vi "Demo RGB LED - Chaser With R G B Alternate onboard LED.vi"   [LabVIEW 2015]
doc: "This example demonstrates a theater light chaser on a 1-wire RGB LED strip using a WS2811 or WS2812 controller. The color of all LEDs can be preset on the front panel as well as the number of lights to cycle in the light chase. The time delay can also be adjusted to change the dramatic effect."
uses:
  <vilib>/Aledyne-TSXperts/Arduino Compatible Compiler for LabVIEW/Code Generator/Arduino APIs/Digital/PinDirection.ctl
  <vilib>/Aledyne-TSXperts/Arduino Compatible Compiler for LabVIEW/Code Generator/Arduino APIs/RGB LED Strip/RGB Strip Mode.ctl
  LED State.vi
  <vilib>/Aledyne-TSXperts/Arduino Compatible Compiler for LabVIEW/Arduino Compatible Compiler for LabVIEW.lvlib
panel:
  # "Overview: Demonstrates a theater light chaser on a 1-wire RGB LED strip using a WS2811 or WS2812 controller.  The color of all LEDs can be preset as well as the number of lights to cycle in the light chase.  The time delay can also be adjusted to change the dramatic effect.\n\nInstructions:\n1. Wire a 1-wire LED strip to a digital pin on the Arduino board.  Follow wiring instructions from the manufacturer.  A 100-500 ohm resistor is usually recommended between the Arduino digital output and the LED strip's data in pin.  Also, a 100 uF capacitor between the ground and power input may reduce noise on from the power supply.  It is also recommended to power the LED strip from a separate power input if available on the strip.  When daisy chaining LED strips, it is recommended to only daisy chain the Data line and to power each strip from a separate power input.\n2. Set the Digital Pin wired below.\n3. Set the Mode to the correct setting for your LED strip (the WS2812 uses 800kHz GRB).\n4. Set the Number of LEDs on your strip.  This can be set to any number equal to or smaller than the number of physical LEDs on the strip of you do not wish to power up all of them.\n5. Set Chase Every N Pixel to adjust how many pixels are moved on every cycle.\n6. Set the delay (ms) between LED rotations/shifts.\n7. Set the Red, Blue, and Green color of all LEDs on the strip.\n8.  If this example has been loaded from the Arduino Compatible Compiler for LabVIEW, simply select Compile and Download.  Otherwise, open Tools>Arduino Compatible Compiler for LabVIEW in LabVIEW, then select File>Load VI, and select this VI and then Compile and Download.\n9. Observe the LEDs on the strip as they appear to chase each other down the strip in a linear movement."
types:
  T1 = typedef "Arduino Compatible Compiler for LabVIEW.lvlib/RGB Strip Mode.ctl" = u16
  T2 = typedef "Arduino Compatible Compiler for LabVIEW.lvlib/PinDirection.ctl" = enum16{" INPUT", "OUTPUT", " INPUT_PULLUP"}
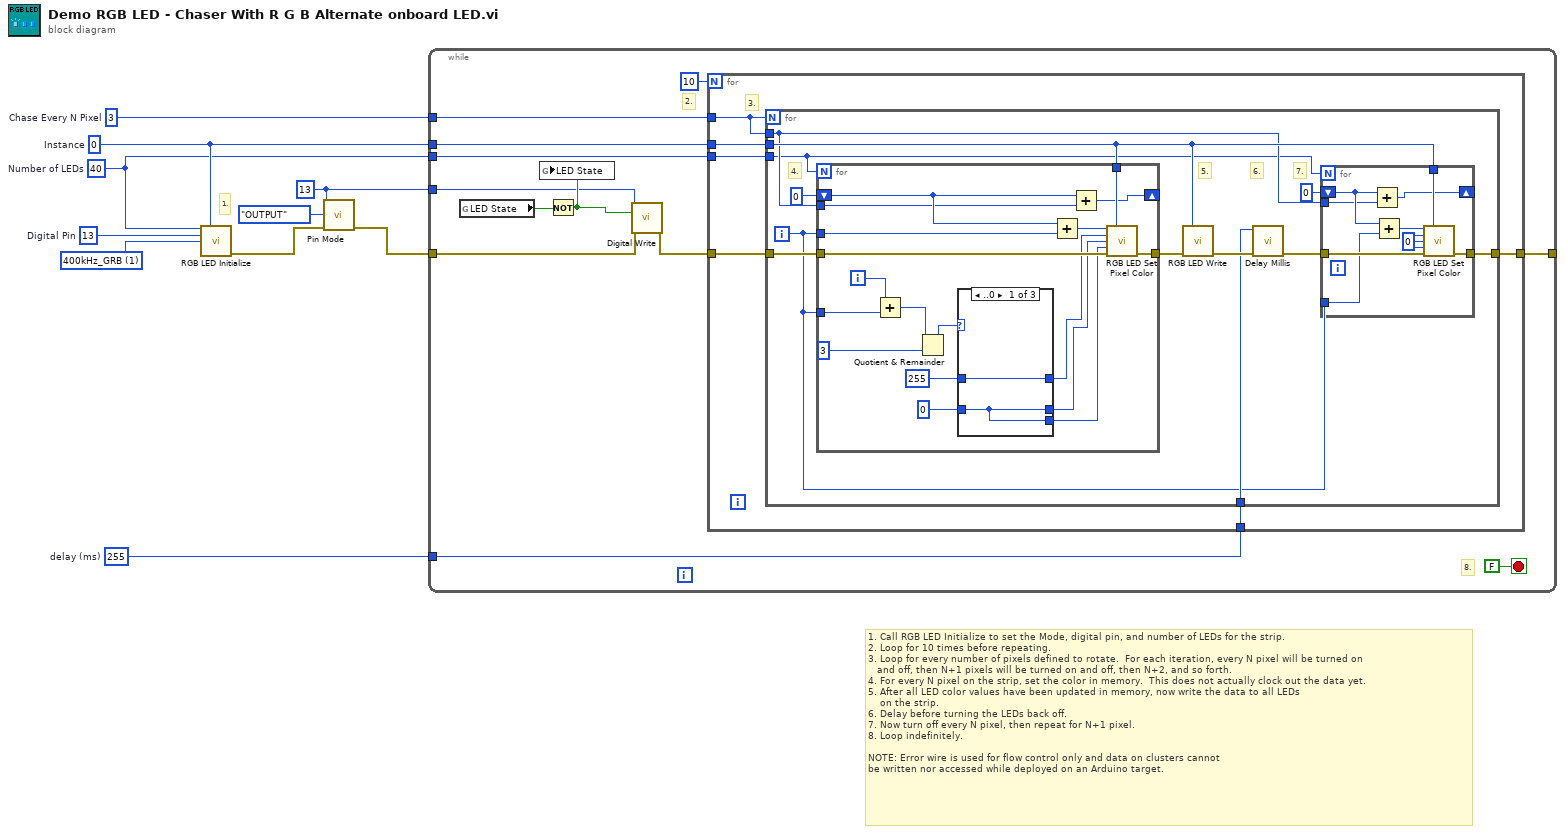
[diagram p0: block diagram]
diagram:
  w5 = u8 255  # delay (ms)
  w10 = T1 1 items=["400kHz_RGB"=0, "400kHz_GRB"=1, "400kHz_BRG"=4, "800kHz_RGB"=2, "800kHz_GRB"=3, "400kHz_BRG"=6] ("Mode")
  w9 = u8 13  # Digital Pin
  w6 = u16 40  # Number of LEDs
  w7 = u8 3  # Chase Every N Pixel
  w1 = u8 13 ("pin")
  w8 = u8 0  # Instance
  # "1."
  # "1. Call RGB LED Initialize to set the Mode, digital pin, and number of LEDs for the strip.\n2. Loop for 10 times before repeating.\n3. Loop for every number of pixels defined to rotate.  For each iteration, every N pixel will be turned on\n   and off, then N+1 pixels will be turned on and off, then N+2, and so forth.\n4. For every N pixel on the strip, set the color in memory.  This does not actually clock out the data yet. \n5. After all LED color values have been updated in memory, now write the data to all LEDs\n    on the strip.\n6. Delay before turning the LEDs back off.\n7. Now turn off every N pixel, then repeat for N+1 pixel.\n8. Loop indefinitely.\n\nNOTE: Error wire is used for flow control only and data on clusters cannot\nbe written nor accessed while deployed on an Arduino target."
  n1 = call <vilib>:"RGB LED Initialize.vi"("Number of Pixels"=w6, "Instance"=w8, "Pin"=w9, "Mode"=w10) -> ("error out"=w4:errorcluster)  [unwired: 11 in]
  n2 = call <vilib>:"Pin Mode.vi"("pin"=w1, "direction"=PinDirection."OUTPUT", "error in (no error)"=w4) -> ("error out"=w3:errorcluster)  [unwired: 12 in]
  n3 = while {
    tunnel: w3 -> [w12]
    tunnel: w8 -> [w20]
    tunnel: w7 -> [w19]
    tunnel: w6 -> [w18]
    tunnel: [w17] -> _
    tunnel: w5 -> [w16]
    tunnel: w1 -> [w13]
    stop <- FALSE stop-if-true
    # "8."
    # "2."
    n4 = global read "LED State.vi" "LED State"() -> (w15:bool)
    n5 = Not(x=w15) -> (.not. x?=w14:bool)
    n6 = global write "LED State.vi" "LED State"(w14) -> ()
    n7 = call <vilib>:"Digital Write.vi"("pin"=w13, "state"=w14, "error in (no error)"=w12) -> ("error out"=w11:errorcluster)  [unwired: 12 in]
    n8 = for {
      N: u16 10 ("Number of Pixels") -> [_]
      tunnel: w20 -> [w28]
      tunnel: w11 -> [w27]
      tunnel: w19 -> [w26]
      tunnel: w18 -> [w25]
      tunnel: [w24] -> w17
      tunnel: w16 -> [w23]
      # "3."
      n9 = for {
        N: w26 -> [_]
        tunnel: w28 -> [w36]
        tunnel: w27 -> [w39]
        tunnel: w26 -> [w33]
        tunnel: w25 -> [w32]
        tunnel: [w31] -> w24
        tunnel: w23 -> [w30]
        i -> [w29]
        # "7."
        # "6."
        # "5."
        # "4."
        n10 = for {
          N: w32 -> [_]
          tunnel: w36 -> [w67]
          tunnel: w29 -> [w66]
          tunnel: [w65] -> w40
          tunnel: w39 -> [w64]
          shift-right: [w63] -> _
          shift-left: u8 0 ("Number of Pixels") -> [w61]
          tunnel: w33 -> [w60]
          tunnel: w29 -> [w52]
          i -> [w51]
          n11 = Add(x=w51, y=w52) -> (x+y=w50:i32)
          n12 = Quotient & Remainder(x=w50, y=3) -> (x-y*floor(x/y)=w58:i32)  [unwired: 1 out]
          n13 = case shown="..0" w58 {
            tunnel: u8 255 ("Red") -> [w69 w70 w72]
            tunnel: [w69 w71 w73] -> w56
            tunnel: u8 0 ("Red") -> [w68 w71 w73]
            tunnel: [w68 w70 w73] -> w54
            tunnel: [w68 w71 w72] -> w53
            frame ..0 {
            }
            frame 1 {
            }
            frame 2.. {
            }
          }
          n14 = Add(x=w61, y=w66) -> (x+y=w62:i32)
          n15 = Add(x=w61, y=w60) -> (x+y=w63:u8)
          n16 = call <vilib>:"RGB LED Set Pixel Color.vi"("Pixel"=w62, "Instance"=w67, "Red"=w56, "Green"=w54, "Blue"=w53, "error in (no error)"=w64) -> ("error out"=w65:errorcluster)  [unwired: 9 in]
        }
        n17 = call <vilib>:"RGB LED Write.vi"("Instance"=w36, "error in (no error)"=w40) -> ("error out"=w38:errorcluster)  [unwired: 13 in]
        n18 = call <vilib>:"Delay Millis.vi"("error in (no error)"=w38, "delay"=w30) -> ("error out"=w37:errorcluster)  [unwired: 9 in]
        n19 = for {
          N: w32 -> [_]
          tunnel: w36 -> [w49]
          tunnel: [w47] -> w31
          tunnel: w37 -> [w46]
          tunnel: w29 -> [w44]
          shift-right: [w43] -> _
          shift-left: u8 0 ("Number of Pixels") -> [w42]
          tunnel: w33 -> [w41]
          w45 = u8 0 ("Red")
          n20 = Add(x=w42, y=w41) -> (x+y=w43:u8)
          n21 = Add(x=w42, y=w44) -> (x+y=w48:i32)
          n22 = call <vilib>:"RGB LED Set Pixel Color.vi"("Pixel"=w48, "Instance"=w49, "Red"=w45, "Green"=w45, "Blue"=w45, "error in (no error)"=w46) -> ("error out"=w47:errorcluster)  [unwired: 9 in]
        }
      }
    }
  }
